vi "PasswordPrompt.vi"() -> (2 "Please enter password below 2":string)   [LabVIEW 2020]
panel:
  in  "OK Button":bool
  in  "Please enter password below":string
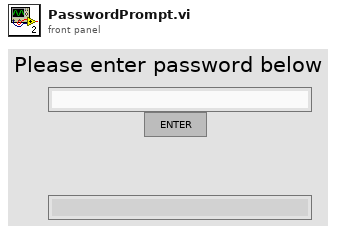
[diagram p1: front panel]
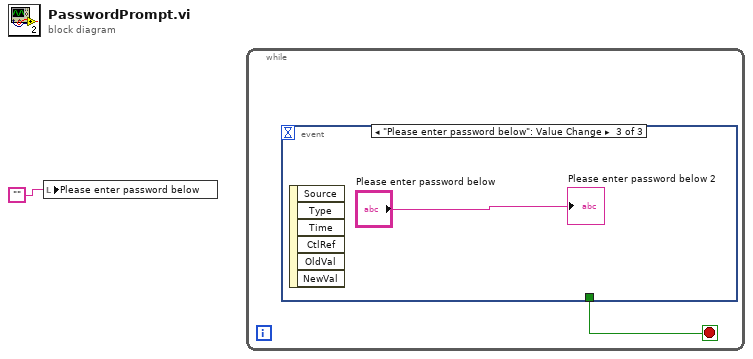
[diagram p0: block diagram]
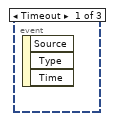
[diagram p2: hidden frame]
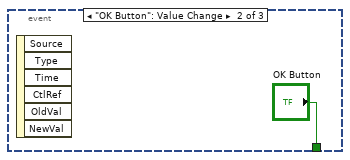
[diagram p3: hidden frame]
diagram:
  n1 = local write "Please enter password below"("") -> ()
  n2 = while {
    stop <- w2 stop-if-true
    n3 = event shown="[2] \"Please enter password below\": Value Change" {
      selector: _ -> [_ _ _]
      dyn-events: _ -> [_ _ _]
      timeout: _ -> [_ _ _]
      tunnel: [_ "OK Button" _] -> w2
      event Timeout {
        n4 = event-data() -> ()  [unwired: 1 in, 3 out]
      }
      event "OK Button": Value Change {
        n5 = event-data() -> ()  [unwired: 1 in, 6 out]
      }
      event "Please enter password below": Value Change {
        n6 = event-data() -> ()  [unwired: 1 in, 6 out]
        "Please enter password below 2" <- "Please enter password below"
      }
    }
  }
